vi "offline analyzer.vi"() -> ()   [LabVIEW 2017]
uses:
  <vilib>/Utility/file.llb/Read Delimited Spreadsheet (I64).vi
panel:
  in  "通道数量":i32=128
  in  "codeDensity":path=path "G:/tdc/2017/test_20240327_123704_codeDensity.csv"
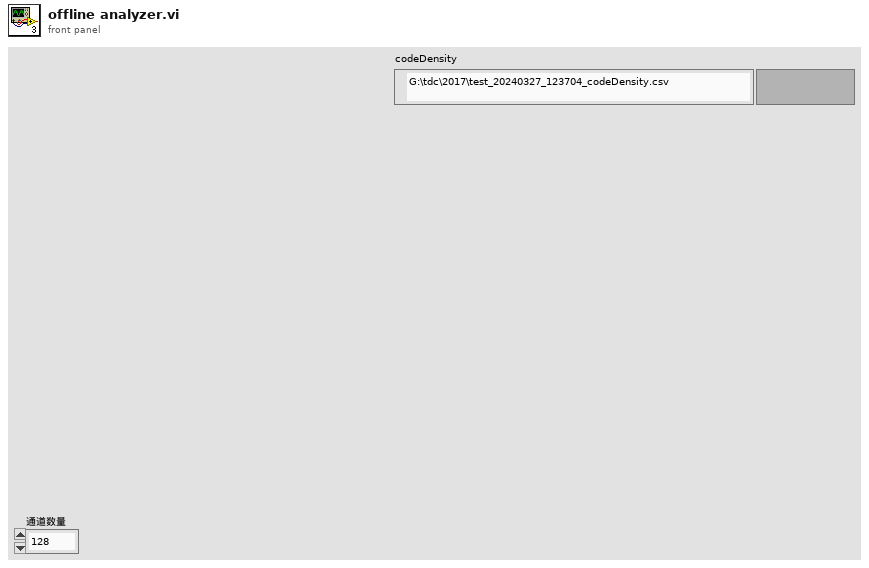
[diagram p1: front panel]
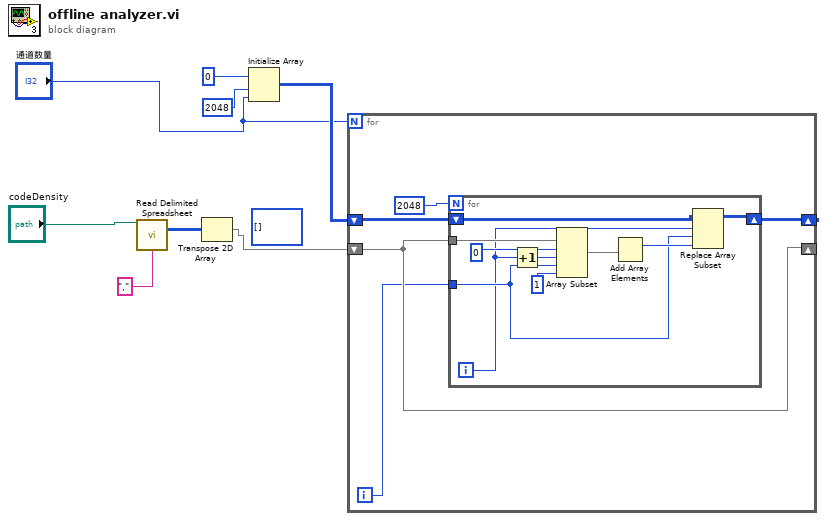
[diagram p0: block diagram]
diagram:
  (unwired) i64[][] []
  n1 = call-poly <vilib>:"Read Delimited Spreadsheet.vi"("file path (dialog if empty)"="codeDensity", "delimiter (\\t)"="," ("delimiter (\\t)")) -> ("all rows"=w8:i64[][])  [unwired: 8 in, 5 out]
  n2 = Transpose 2D Array(2D array=w8) -> (transposed array=w2:i64[][])
  n3 = Initialize Array(u32 0 ("element"), 2048 ("dimension size"), "通道数量") -> (w3:u32[][])
  n4 = for {
    N: "通道数量" -> [_]
    shift-right: [w11] -> _
    shift-left: w3 -> [w12]
    shift-right: [w10] -> _
    shift-left: w2 -> [w10]
    i -> [w9]
    n5 = for {
      N: 2048 -> [_]
      tunnel: w10 -> [w23]
      tunnel: w9 -> [w16]
      shift-right: [w18] -> w11
      shift-left: w12 -> [w19]
      i -> [w15]
      n6 = Increment(x=w15) -> (x+1=w14:i32)
      n7 = Array Subset(array=w23, index (row)=0 ("索引"), length (row)=w14, index (col)=w16, length (col)=1 ("长度")) -> (w20:i64[][])
      n8 = Add Array Elements(numeric array=w20) -> (sum=w17:i64)
      n9 = Replace Array Subset(array=w19, new element=w17, index (row)=w15, index (col)=w16) -> (w18:u32[][])
    }
  }
